vi "Field Get MN SN Display Names.vi"(8 "error in (no error)":errorcluster, 11 "Connection Refnum":T1) -> (0 "error out":errorcluster, 1 "Serial Number Display Name":string, 2 "Model Number Display Name":string, 3 "Connection Refnum":T1)   [LabVIEW 2011]
uses:
  SI.LIB/ODBC/SQL Controls/Connection Refnum.ctl
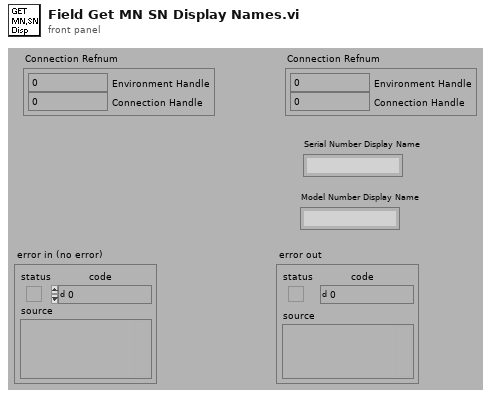
[diagram p1: front panel]
types:
  T1 = typedef "Connection Refnum.ctl" = cluster{"Environment Handle":i32, "Connection Handle":i32}
  T2 = typedef "Field Record.ctl" = cluster{"ixField":i32, "iSequenceOrder":i32, "sxFieldId":string, "sxSequenceId":string, "sDisplayName":string, "sValue":string, "sUnits":string, "nDataType":T3, "nNextItem":T4, "fSystem":bool, "fSystemValue":bool, "fRequired":bool, "fSetAtTest":bool, "fTestField":bool, "fDeleted":bool, "fIndexed":bool, "fFreeList":bool}
  T3 = typedef "Field DataTypes.ctl" = enum32{"text", "numeric", "list", "timestamp", "boolean"}
  T4 = typedef "Field NextItem.ctl" = enum32{"Reset", "Retain", "Auto-Increment"}
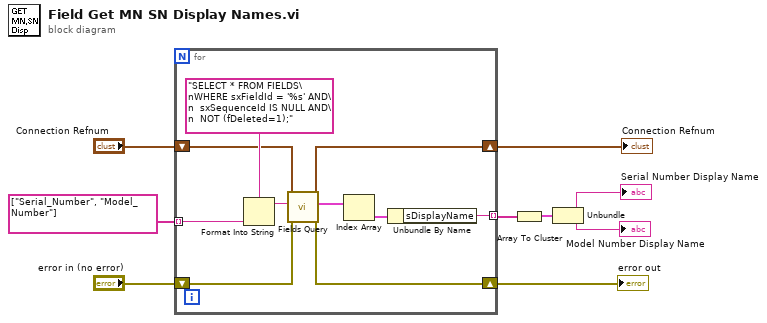
[diagram p0: block diagram]
diagram:
  n1 = for {
    tunnel: string[] ["Serial_Number", "Model_Number"] -> [w16] mode=indexing
    shift-right: [w12] -> w5
    shift-left: "Connection Refnum" -> [w13]
    shift-right: [w14] -> w6
    shift-left: "error in (no error)" -> [w15]
    tunnel: [w10] -> w4 mode=indexing
    n2 = Format Into String(format string="SELECT * FROM FIELDS\nWHERE sxFieldId = '%s' AND\n  sxSequenceId IS NULL AND\n  NOT (fDeleted=1);" ("Query Name"), w16) -> (resulting string=w11:string)  [unwired: 2 in, 1 out]
    n3 = call "Fields Query.vi"("error in (no error)"=w15, "Query"=w11, "Connection Refnum"=w13) -> ("error out"=w14:errorcluster, "Fields"=w19:T2[], "Connection Refnum"=w12:T1)  [unwired: 1 in, 5 out]
    n4 = Index Array(array=w19) -> (element=w18:T2)  [unwired: 1 in]
    n5 = Unbundle By Name(w18) -> ("sDisplayName"=w10:string)
  }
  "error out" <- w6
  "Connection Refnum" <- w5
  n6 = Array To Cluster(array=w4) -> (cluster=w3:cluster{"[0]":string, "[1]":string})
  n7 = Unbundle(w3) -> ("[0]"=→"Serial Number Display Name":string, "[1]"=→"Model Number Display Name":string)
